vi "TSM Relay Connections to Configuration Array.vi"(0 "TSM Context":T6, 5 "Relay/Action Connections":T4[][](array[typedef]) {"Relay Action" items=["Open Relay"=20, "Close Relay"=21]}, 9 "TSM Site Numbers":i32[](array[numeric]), 11 "error in":errorcluster) -> (4 "TSM Relay Configuration Array":T1[](array[typedef]) {"SSC Relay with Action"."Relay Action" items=["Open Relay"=20, "Close Relay"=21]}, 15 "error out":errorcluster)   [LabVIEW 2019]
doc: "Populates the TSM Relay Configuration cluster for the selected relay/action connections. This VI can be used to implement a relay configuration (set of mappings between relays and positions) within a test code module. \n\nUse this VI in place of TSM Relay Conections to Configuration VI when optimizing for test time - this allows users to call Get Site Numbers only once in their code module and reduce the number of TSM context calls."
uses:
  <vilib>/NI_TestStand_SemiconductorModule/NI_TestStand_Semiconductor_Module.lvlibp/PinMap/General/SemiconductorModuleContext.ctl
  Pin Map/TSM Relay to Action Map.ctl
  <vilib>/NI_TestStand_SemiconductorModule/NI_TestStand_Semiconductor_Module.lvlibp/1abvi3w/instr.lib/niSwitch/niswitch.llb/niSwitch Relay Action.ctl
  SubVIs/TSM Relay Config.ctl
  <vilib>/NI_TestStand_SemiconductorModule/NI_TestStand_Semiconductor_Module.lvlibp/PinMap/PinQueryContext/MultiplePinMultipleSessionQueryContext/MultiplePinMultipleSessionQueryContext.lvclass
  SSC/SSC Relay.ctl
  <instrlib>/niSwitch/niSwitch.llb/niSwitch Relay Action.ctl
  SubVIs/TSM Relay Configuration Relay Actions to Sessions.vi
  TSM Relay Pins to Sessions.vi
  <vilib>/NI_TestStand_SemiconductorModule/NI_TestStand_Semiconductor_Module.lvlibp
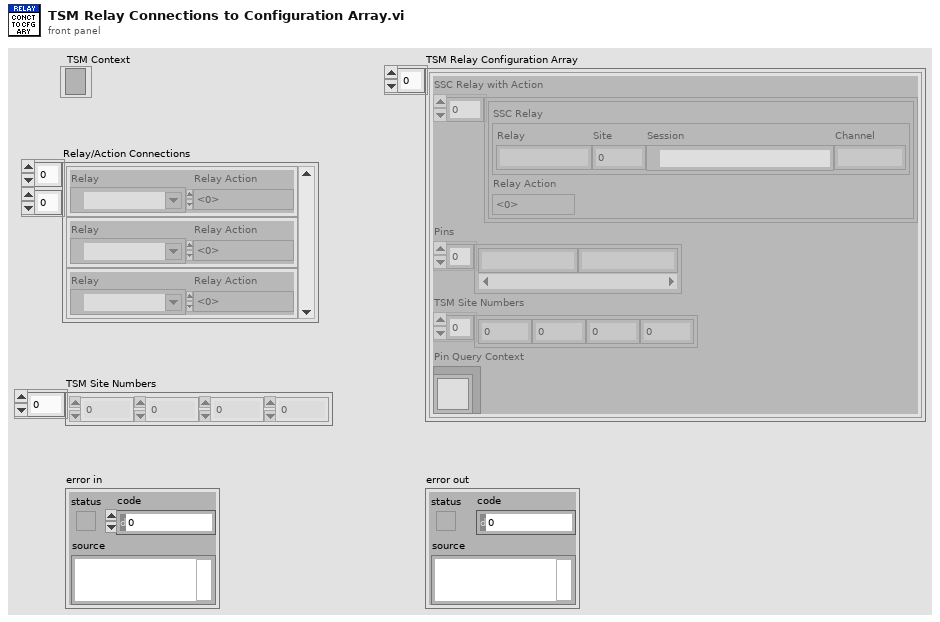
[diagram p1: front panel]
types:
  T1 = typedef "TSM Relay Config.ctl" = cluster{"SSC Relay with Action":cluster{"SSC Relay":T2, "Relay Action":T3}[], "Pins":string[], "TSM Site Numbers":i32[], "Pin Query Context":refnum<class "MultiplePinMultipleSessionQueryContext.lvclass">}
  T2 = typedef "SSC Relay.ctl" = cluster{"Relay":string, "Site":i32, "Session":refnum<k15>, "Channel":string}
  T3 = typedef "niSwitch Relay Action.ctl" = i32
  T4 = typedef "TSM Relay to Action Map.ctl" = cluster{"Relay":tag, "Relay Action":T5}
  T5 = typedef "NI_TestStand_Semiconductor_Module.lvlibp/niSwitch Relay Action.ctl" = i32
  T6 = typedef "NI_TestStand_Semiconductor_Module.lvlibp/SemiconductorModuleContext.ctl" = refnum<k7>
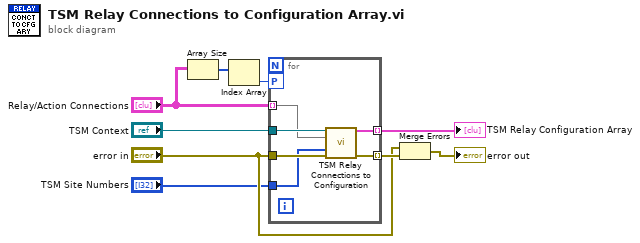
[diagram p0: block diagram]
diagram:
  n1 = Array Size(array="Relay/Action Connections") -> (size(s)=w2:i32[])
  n2 = Index Array(array=w2) -> (element=w1:i32)  [unwired: 1 in]
  n3 = for {
    tunnel: "TSM Context" -> [w13]
    tunnel: "Relay/Action Connections" -> [w12] mode=indexing
    tunnel: "TSM Site Numbers" -> [w10]
    tunnel: [w11] -> w7 mode=indexing
    tunnel: "error in" -> [w14]
    tunnel: [w15] -> w9 mode=indexing
    workers-P: w1 -> [_]
    n4 = call "TSM Relay Connections to Configuration.vi"("TSM Context"=w13, "Relay/Action Connections"=w12, "TSM Site Numbers"=w10, "error in"=w14) -> ("TSM Relay Configuration"=w11:T1, "error out"=w15:errorcluster)  [unwired: 10 in]
  }
  "TSM Relay Configuration Array" <- w7
  n5 = Merge Errors("error in", w9) -> (→"error out":errorcluster)
